vi "Error Processor.vi"(8 "error in (no error)":errorcluster, 11 "New uService Template in":refnum<class "Waiter.lvclass">) -> (0 "error out":errorcluster, 3 "New uService Template out":refnum<class "Waiter.lvclass">)   [LabVIEW 2020, in "Waiter.lvlib" / "Waiter.lvclass"]
doc: "Use this VI to process all the error that are solvable inside this specific uService. Whatever is not possible to process, let it leave this VI and it will be processed by the Error Manager of the Distributed System."
uses:
  Waiter.lvclass
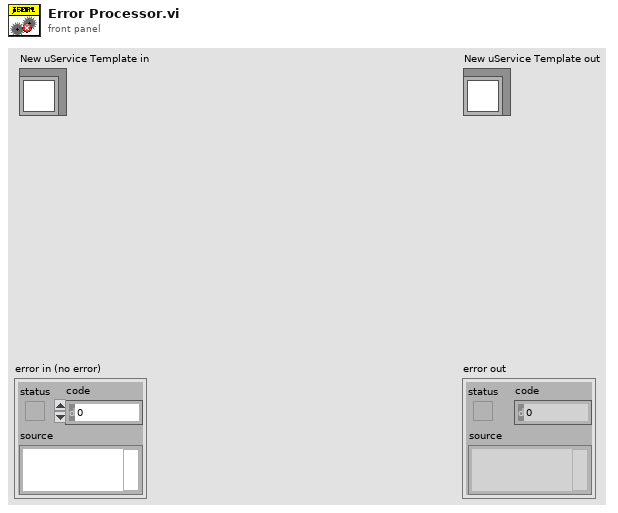
[diagram p1: front panel]
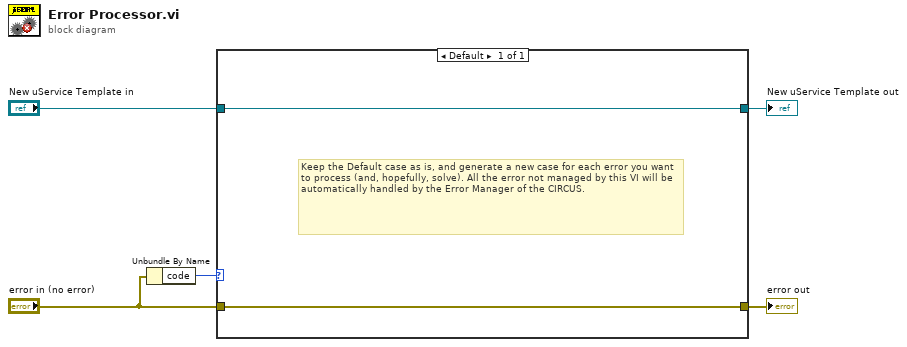
[diagram p0: block diagram]
diagram:
  n1 = Unbundle By Name("error in (no error)") -> ("code"=w2:i32)
  n2 = case shown="Default" w2 {
    tunnel: "New uService Template in" -> [w7]
    tunnel: [w7] -> w4
    tunnel: "error in (no error)" -> [w6]
    tunnel: [w6] -> w1
    frame Default {
      # "Keep the Default case as is, and generate a new case for each error you want to process (and, hopefully, solve). All the error not managed by this VI will be automatically handled by the Error Manager of the CIRCUS."
    }
  }
  "error out" <- w1
  "New uService Template out" <- w4
